vi "Channel Subpanel.vi"() -> ()   [LabVIEW 2021, in "CIF Manager UI.lvlib"]
uses:
  CIF Manager UI.lvlib
  CIFManagerUI Class/Typedef/Channel Connection.ctl
  CIFManagerUI Class/Typedef/Class Data for Manager SubPanel.ctl
  <vilib>/gRPC/LabVIEW gRPC Library/Shared/grpcId.ctl
  <vilib>/CIF Foundation/CIF Core/CIFUI/Typedef/Core UI References.ctl
  <vilib>/CIF Foundation/CIF Core/CIFUI/Typedef/Run Listen Button.ctl
  <vilib>/CIF Foundation/CIF Core/CIFUI/Typedef/SubPanel Events.ctl
  <vilib>/CIF Foundation/CIF Core/CIFUI/Typedef/New Connection Event Data.ctl
  <vilib>/CIF Foundation/CIF Core/CIFUI/Typedef/New Connection Plugin Event Data.ctl
  CIFManagerUI Class/Typedef/Core Manager UI References.ctl
  CIFManagerUI Class/Typedef/New Plugin.ctl
  CIFManagerUI Class/Typedef/CIF_Manager_UI_Tab.ctl
  CIFManagerUI Class/CIF_Manager_UI.lvclass/CIF_Manager_UI.ctl
  <vilib>/CIF Foundation/CIF Core/CIFUI/CIF_UI.lvclass/CIF_UI.ctl
  <vilib>/CIF Foundation/CIF Core/CIFUI/Typedef/Direction to Include.ctl
  <vilib>/CIF Foundation/CIF Utilities/DataTypes/Typedef/Endian.ctl
  <vilib>/CIF Foundation/CIF Core/CIFUI/Typedef/Force Channel.ctl
  <vilib>/CIF Foundation/CIF Core/CIFUI/Utilities/Get Human Readable Error.vi
  <vilib>/CIF Foundation/CIF Utilities/Errors/Append Error Location.vi
  <vilib>/CIF Foundation/CIF Core/CIFUI/Accessors/Read Instrument Studio.vi
  CIFManagerUI Class/CIF_Manager_UI.lvclass
  C:/Program Files/National Instruments/LabVIEW 2021/vi.lib/CIF Foundation/CIF Core/CIFUI/CIF_UI.lvclass
  <vilib>/CIF Foundation/CIF Core/CIFUI/UI Helpers/UI Element Update/Empty Tree by Reference.vi
  CIFManagerUI Class/Manager Functions/SubVIs/Initialize Manager Tab by Reference.vi
  <vilib>/CIF Foundation/CIF Utilities/Errors/Human Readable Error Message.vi
  <vilib>/CIF Foundation/CIF Core/CIFUI/CIF_UI.lvclass
  <vilib>/CIF Foundation/CIF Utilities/DataTypes/DataTypes_CIF_U.lvlib
  <vilib>/gRPC/LabVIEW gRPC Library/grpc-lvsupport-release.lvlib
panel:
  in  "Class Data for Manager SubPanel":T1
  in  "String Force":string
  in  "Force Active":bool
  in  "I64 Force":i64
  in  "U64 Force":u64
  in  "Double Force":dbl
  in  "Forced Data":string
  in  "Channel":string
  in  "Force Channel":bool
  in  "Link Channel":bool
  in  "Connection":T6
  in  "Publisher Channels":string(tree)
  in  "Subscriber Channels":string(tree)
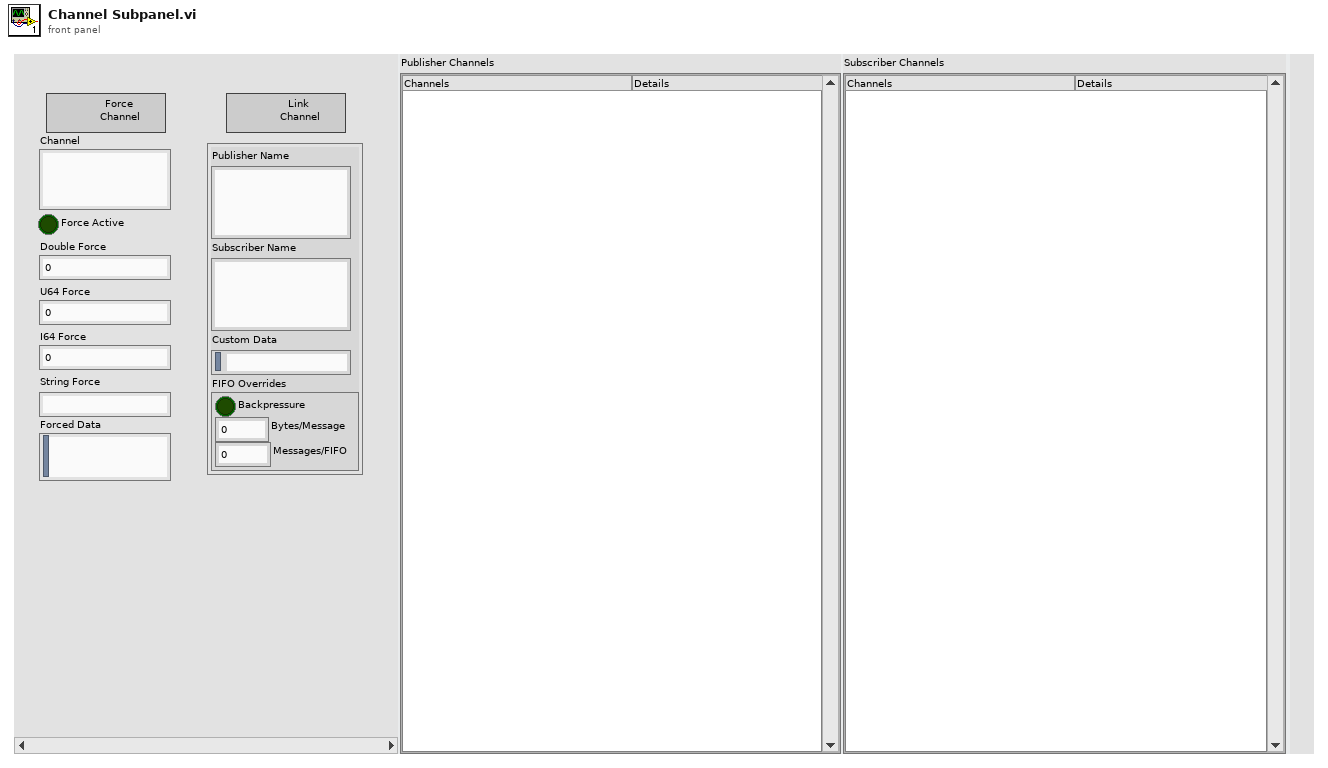
[diagram p1: front panel]
types:
  T1 = typedef "CIF_Manager_UI.lvclass/Class Data for Manager SubPanel.ctl" = cluster{"Class Data for SubPanel":cluster{"IP Address":string, "Manager gRPC ID":T2, "Server Certificate File (.crt)":path, "Connected":bool, "Manager Connection":bool, "Core UI References":T3, "Subpanel Events":T4}, "Manager UI References":T5}
  T2 = typedef "grpc-lvsupport-release.lvlib/grpcId.ctl" = u64
  T3 = typedef "CIF_UI.lvclass/Core UI References.ctl" = cluster{"Plugin Status":refnum<vi>, "Plugin Status Valid":bool, "Connection":refnum<vi>, "Connection Valid":bool, "Exit":refnum<vi>, "Exit Valid":bool, "Run Listen":refnum<vi>, "Run Listen Valid":bool, "Clear Local Error":refnum<vi>, "Clear Local Error Valid":bool, "Local Error":refnum<vi>, "Local Error Valid":bool}
  T4 = typedef "CIF_UI.lvclass/SubPanel Events.ctl" = cluster{"Clear Local Error":refnum<user-event>, "Shutdown":refnum<user-event>, "gRPC Connection":refnum<user-event>, "Plugin Connection":refnum<user-event>}
  T5 = typedef "CIF_Manager_UI.lvclass/Core Manager UI References.ctl" = cluster{"Discovered Plugins":refnum<vi>, "Discovered Plugins Valid":bool, "Loaded Plugins":refnum<vi>, "Loaded Plugins Valid":bool, "Publisher Channels":refnum<vi>, "Publisher Channels Valid":bool, "Subscriber Channels":refnum<vi>, "Subscriber Channels Valid":bool, "Channel Connection":refnum<vi>, "Channel Connection Valid":bool, "New Plugin Load":refnum<vi>, "New Plugin Load Valid":bool, "Errors":refnum<vi>, "Errors Valid":bool, "Plugin to Abort":refnum<vi>, "Plugin to Abort Valid":bool, "CIF Manager Tab":refnum<vi>, "Manger Tab Valid":bool, "System Errors":refnum<vi>, "System Errors Valid":bool, "Plugin Selection":refnum<vi>, "Plugin Selection Valid":bool}
  T6 = typedef "CIF_Manager_UI.lvclass/Channel Connection.ctl" = cluster{"Publisher Name":string, "Subscriber Name":string, "Custom Data":string, "FIFO Overrides":cluster{"Backpressure":bool, "Bytes/Message":u32, "Messages/FIFO":u32}}
  T7 = typedef "CIF_UI.lvclass/Direction to Include.ctl" = enum16{"All", "Subscriber", "Publisher"}
  T8 = enum16{"big-endian, network order", "native, host order", "little-endian"}
  T9 = typedef "DataTypes_CIF_U.lvlib/Endian.ctl" = enum16{"Little Endian", "Big Endian"}
  T10 = typedef "CIF_UI.lvclass/Force Channel.ctl" = cluster{"channel_name":string, "force":bool, "force_data":string}
  T11 = typedef "CIFCoreChannel_client.lvlib/cif_management_common_Channel.ctl" = cluster{"name":string, "direction":T12, "type":string, "custom_config":u8[], "connected":bool, "connected_name":string, "forced":bool, "channel_pattern":T13}
  T12 = typedef "CIFCoreChannel_client.lvlib/cif_management_common_ChannelDirection.ctl" = enum32{"CHANNELDIRECTION_UNKNOWN", "CHANNELDIRECTION_PUBLISHER", "CHANNELDIRECTION_SUBSCRIBER"}
  T13 = typedef "CIFCoreChannel_client.lvlib/cif_management_common_ChannelPattern.ctl" = enum32{"CHANNELPATTERN_UNKNOWN", "CHANNELPATTERN_TAG", "CHANNELPATTERN_FIFO", "CHANNELPATTERN_MULTIFIFO", "CHANNELPATTERN_BACKPRESSUREFIFO"}
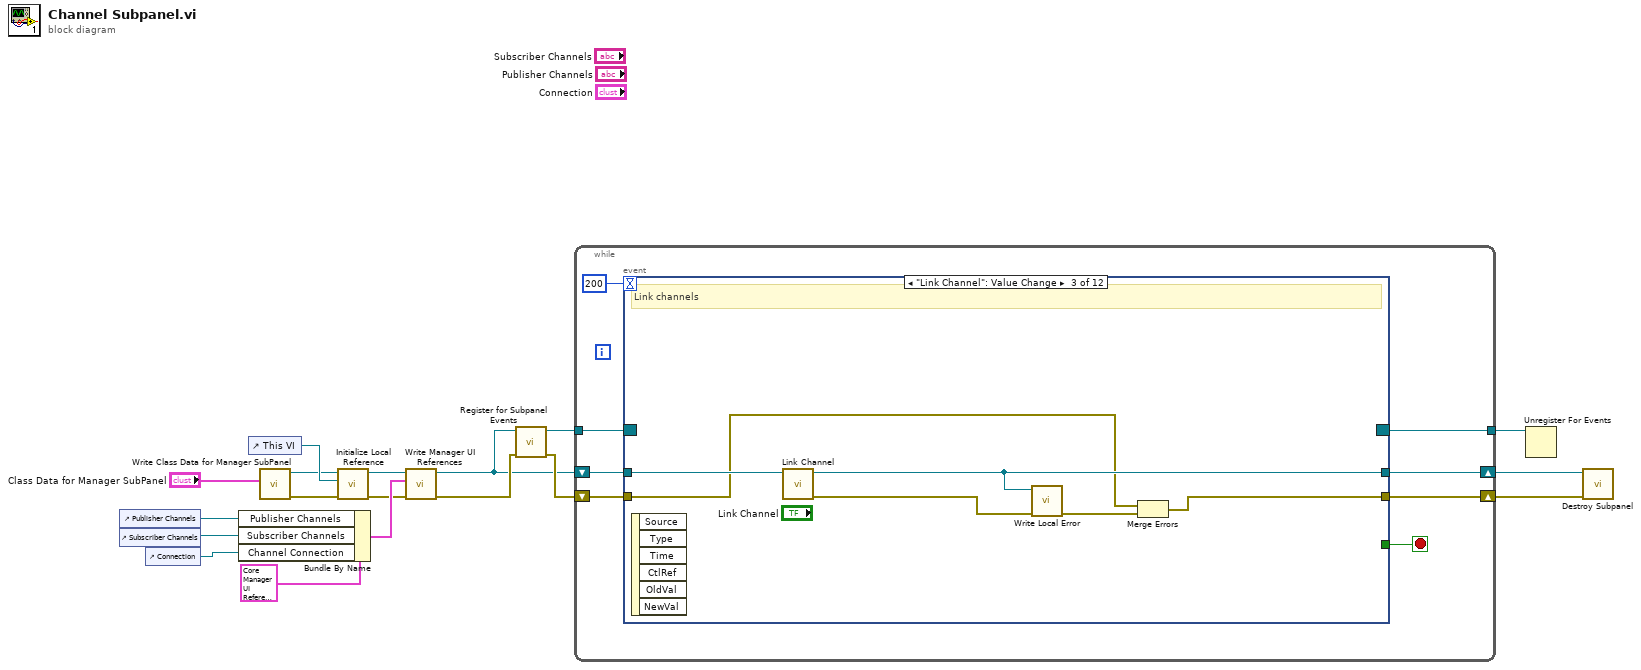
[diagram p0: block diagram]
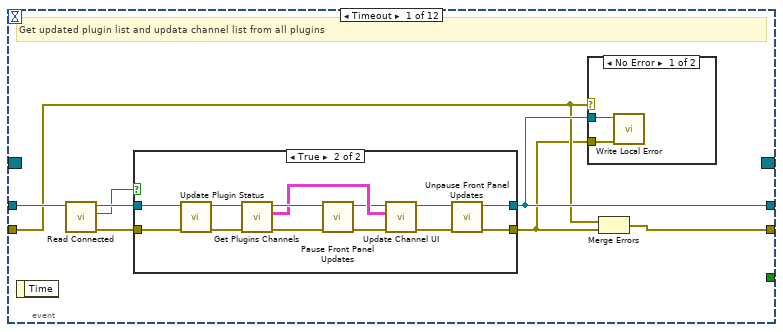
[diagram p2: hidden frame]
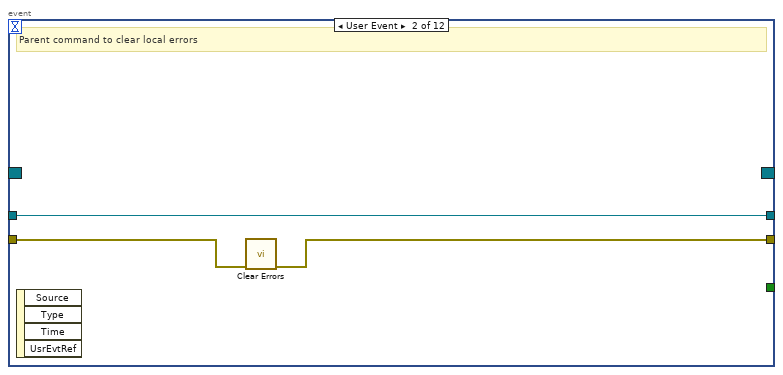
[diagram p5: hidden frame]
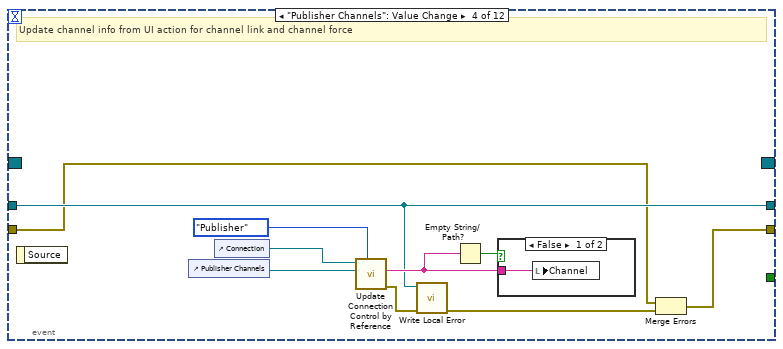
[diagram p6: hidden frame]
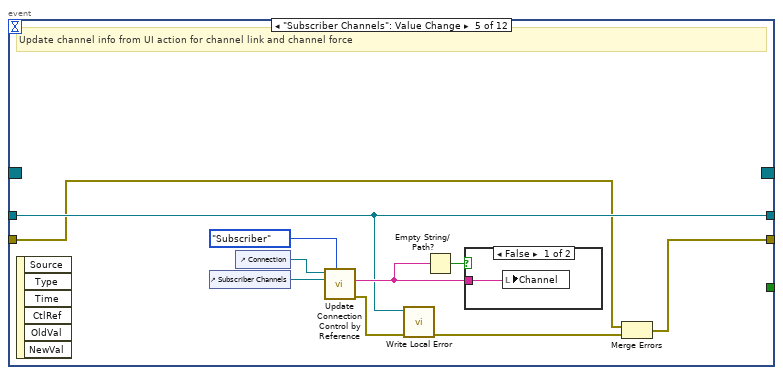
[diagram p8: hidden frame]
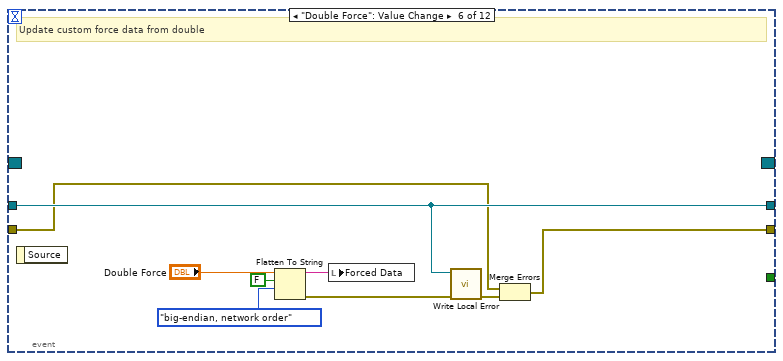
[diagram p10: hidden frame]
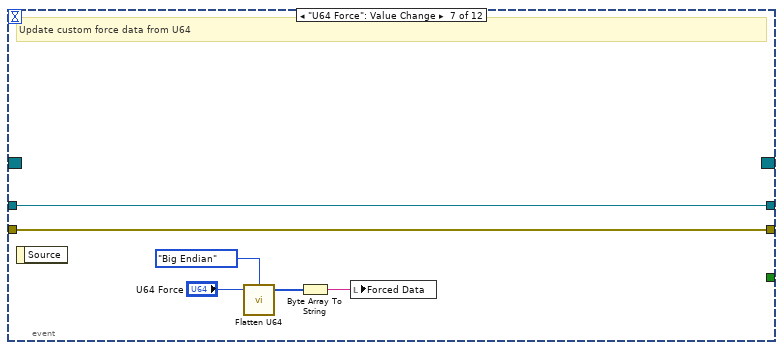
[diagram p11: hidden frame]
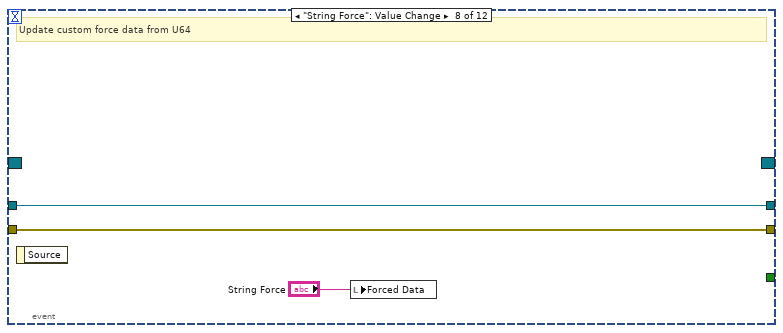
[diagram p12: hidden frame]
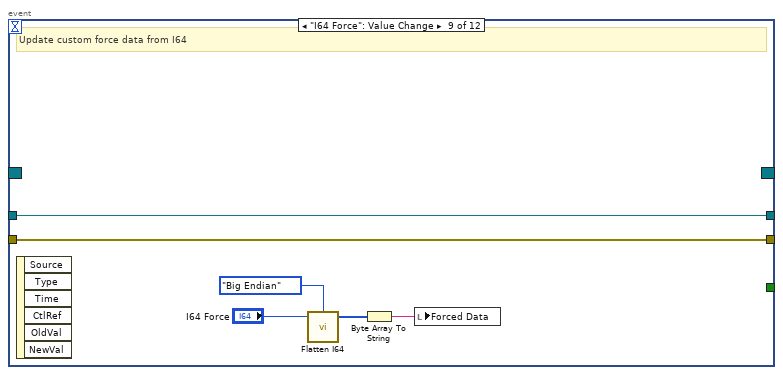
[diagram p13: hidden frame]
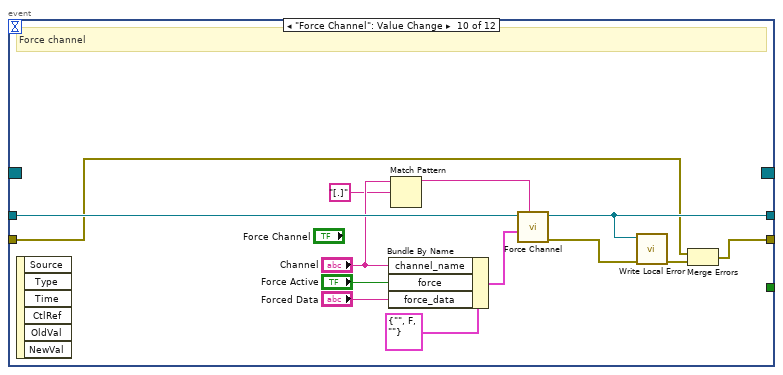
[diagram p14: hidden frame]
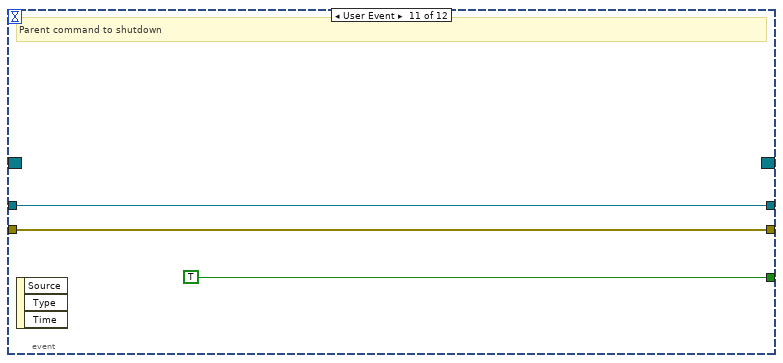
[diagram p15: hidden frame]
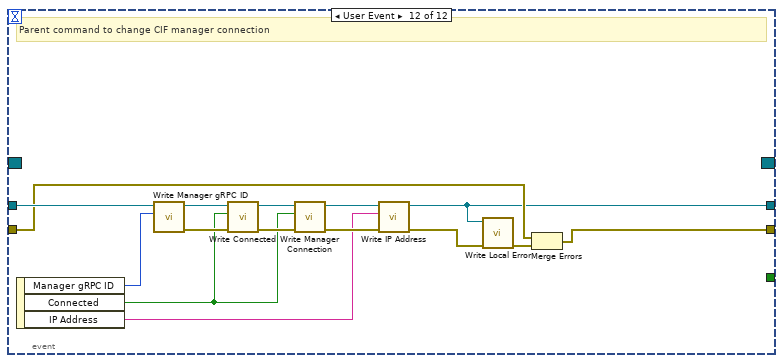
[diagram p16: hidden frame]
diagram:
  n1 = control-ref of="Publisher Channels"() -> (w18:refnum<vi>)
  n2 = control-ref of="Subscriber Channels"() -> (w17:refnum<vi>)
  n3 = control-ref of="Connection"() -> (w16:refnum<vi>)
  n4 = Bundle By Name(cluster=T5 {"Discovered Plugins"=refnum, "Discovered Plugins Valid"=FALSE, "Loaded Plugins"=refnum, "Loaded Plugins Valid"=FALSE, "Publisher Channels"=refnum, "Publisher Channels Valid"=FALSE, "Subscriber Channels"=refnum, "Subscriber Channels Valid"=FALSE, "Channel Connection"=refnum, "Channel Connection Valid"=FALSE, "New Plugin Load"=refnum, "New Plugin Load Valid"=FALSE, "Errors"=refnum, "Errors Valid"=FALSE, "Plugin to Abort"=refnum, "Plugin to Abort Valid"=FALSE, "CIF Manager Tab"=refnum, "Manger Tab Valid"=FALSE, "System Errors"=refnum, "System Errors Valid"=FALSE, "Plugin Selection"=refnum, "Plugin Selection Valid"=FALSE} ("Manager UI References"), "Publisher Channels"=w18, "Subscriber Channels"=w17, "Channel Connection"=w16) -> (w9:T5)
  n5 = control-ref of="This VI"() -> (w13:refnum<vi>)
  n6 = call "Write Class Data for Manager SubPanel.vi"("Class Data for Manager SubPanel"="Class Data for Manager SubPanel") -> ("error out"=w4:errorcluster, "CIF_Manager_UI out"=w3:refnum<class "CIF_Manager_UI.lvclass">)  [unwired: 9 in]
  n7 = call <vilib>:"Initialize Local Reference.vi"("error in (no error)"=w4, "This VI"=w13, "CIF_UI in"=w3) -> ("error out"=w7:errorcluster, "CIF_UI out"=w8:refnum<class "CIF_Manager_UI.lvclass">)  [unwired: 7 in]
  n8 = call "Write Manager UI References.vi"("error in (no error)"=w7, "Manager UI References"=w9, "CIF_UI in"=w8) -> ("error out"=w6:errorcluster, "CIF_UI out"=w5:refnum<class "CIF_Manager_UI.lvclass">)  [unwired: 7 in]
  n9 = call <vilib>:"Register for Subpanel Events.vi"("error in (no error)"=w6, "CIF_UI in"=w5) -> ("error out"=w14:errorcluster, "Event Registration Refnum"=w15:refnum<event-registration>)  [unwired: 8 in]
  n10 = while {
    tunnel: w15 -> [w25]
    shift-right: [w21] -> w12
    shift-left: w5 -> [w23]
    shift-right: [w19] -> w10
    shift-left: w14 -> [w22]
    tunnel: [w20] -> w11
    stop <- w24 stop-if-true
    n11 = event shown="[2] \"Link Channel\": Value Change" {
      selector: w25 -> [_ _ _ _ _ _ _ _ _ _ _ _]
      dyn-events: [_ _ _ _ _ _ _ _ _ _ _ _] -> w20
      timeout: 200 -> [_ _ _ _ _ _ _ _ _ _ _ _]
      tunnel: [_ _ _ _ _ _ _ _ _ _ TRUE _] -> w24
      tunnel: w23 -> [w31 w52 w60 w64 w75 w85 w97 w100 w102 w119 w121 w131]
      tunnel: w22 -> [w29 w54 w56 w62 w72 w84 w96 w99 w101 w107 w120 w124]
      tunnel: [w27 w53 w55 w61 w73 w83 w96 w99 w101 w108 w120 w125] -> w19
      tunnel: [w30 w52 w59 w64 w75 w85 w97 w100 w102 w111 w121 w123] -> w21
      event Timeout {
        # "Get updated plugin list and updata channel list from all plugins"
        n12 = event-data() -> ()  [unwired: 1 in, 1 out]
        n13 = call <vilib>:"Read Connected.vi"("CIF_UI in"=w31) -> ("error out"=w33:errorcluster, "Connected"=w32:bool, "CIF_UI out"=w34:refnum<class "CIF_Manager_UI.lvclass">)  [unwired: 8 in]
        n14 = case shown="True" w32 {
          tunnel: w33 -> [w37 w44]
          tunnel: [w37 w51] -> w28
          tunnel: w34 -> [w38 w45]
          tunnel: [w38 w50] -> w30
          frame False {
          }
          frame True {
            n15 = call <vilib>:"Update Plugin Status.vi"("error in (no error)"=w44, "CIF_UI in"=w45) -> ("error out"=w48:errorcluster, "CIF_UI out"=w49:refnum<class "CIF_Manager_UI.lvclass">)  [unwired: 8 in]
            n16 = call <vilib>:"Get Plugins Channels.vi"("error in (no error)"=w48, "CIF_UI in"=w49) -> ("error out"=w40:errorcluster, "Channels"=w42:T11[][], "CIF_UI out"=w43:refnum<class "CIF_Manager_UI.lvclass">)  [unwired: 6 in, 1 out]
            n17 = call <vilib>:"Pause Front Panel Updates.vi"("error in (no error)"=w40, "CIF_UI in"=w43) -> ("error out"=w39:errorcluster, "CIF_UI out"=w41:refnum<class "CIF_Manager_UI.lvclass">)  [unwired: 8 in]
            n18 = call "Update Channel UI.vi"("error in (no error)"=w39, "Channels"=w42, "CIF_UI in"=w41) -> ("error out"=w46:errorcluster, "CIF_UI out"=w47:refnum<class "CIF_Manager_UI.lvclass">)  [unwired: 7 in]
            n19 = call <vilib>:"Unpause Front Panel Updates.vi"("error in (no error)"=w46, "CIF_UI in"=w47) -> ("error out"=w51:errorcluster, "CIF_UI out"=w50:refnum<class "CIF_Manager_UI.lvclass">)  [unwired: 8 in]
          }
        }
        n20 = case shown="No Error" w29 {
          tunnel: w28 -> [w36 _]
          tunnel: w30 -> [w35 _]
          frame No Error {
            n21 = call <vilib>:"Write Local Error.vi"("error in (no error)"=w36, "CIF_UI in"=w35) -> ()  [unwired: 9 in, 1 out]
          }
          frame Error {
          }
        }
        n22 = Merge Errors(w29, w28) -> (w27:errorcluster)
      }
      event User Event {
        # "Parent command to clear local errors"
        n23 = event-data() -> ()  [unwired: 1 in, 4 out]
        n24 = call <vilib>:"Clear Errors.vi"("error in (no error)"=w54) -> ("error out"=w53:errorcluster)  [unwired: 5 in, 1 out]
      }
      event "Link Channel": Value Change {
        # "Link channels"
        n25 = event-data() -> ()  [unwired: 1 in, 6 out]
        n26 = call "Link Channel.vi"("CIF_UI in"=w60) -> ("error out"=w58:errorcluster, "CIF_UI out"=w59:refnum<class "CIF_Manager_UI.lvclass">)  [unwired: 9 in]
        n27 = call <vilib>:"Write Local Error.vi"("error in (no error)"=w58, "CIF_UI in"=w59) -> ("error out"=w57:errorcluster)  [unwired: 9 in]
        n28 = Merge Errors(w56, w57) -> (w55:errorcluster)
      }
      event "Publisher Channels": Value Change {
        # "Update channel info from UI action for channel link and channel force"
        n29 = event-data() -> ()  [unwired: 1 in, 1 out]
        n30 = control-ref of="Publisher Channels"() -> (w68:refnum<vi>)
        n31 = control-ref of="Connection"() -> (w69:refnum<vi>)
        n32 = call "Update Connection Control by Reference.vi"("Direction to Include"=Direction_to_Include."Publisher", "Channels"=w68, "Channel Connection"=w69) -> ("error out"=w65:errorcluster, "Channel Name"=w66:string)  [unwired: 7 in]
        n33 = call <vilib>:"Write Local Error.vi"("error in (no error)"=w65, "CIF_UI in"=w64) -> ("error out"=w63:errorcluster)  [unwired: 9 in]
        n34 = Empty String/Path?(string/path=w66) -> (empty?=w67:bool)
        n35 = case shown="False" w67 {
          tunnel: w66 -> [w71 _]
          frame False {
            n36 = local write "Channel"(w71) -> ()
          }
          frame True {
          }
        }
        n37 = Merge Errors(w62, w63) -> (w61:errorcluster)
      }
      event "Subscriber Channels": Value Change {
        # "Update channel info from UI action for channel link and channel force"
        n38 = event-data() -> ()  [unwired: 1 in, 6 out]
        n39 = control-ref of="Subscriber Channels"() -> (w79:refnum<vi>)
        n40 = control-ref of="Connection"() -> (w80:refnum<vi>)
        n41 = call "Update Connection Control by Reference.vi"("Direction to Include"=Direction_to_Include."Subscriber", "Channels"=w79, "Channel Connection"=w80) -> ("error out"=w76:errorcluster, "Channel Name"=w77:string)  [unwired: 7 in]
        n42 = call <vilib>:"Write Local Error.vi"("error in (no error)"=w76, "CIF_UI in"=w75) -> ("error out"=w74:errorcluster)  [unwired: 9 in]
        n43 = Empty String/Path?(string/path=w77) -> (empty?=w78:bool)
        n44 = case shown="False" w78 {
          tunnel: w77 -> [w82 _]
          frame False {
            n45 = local write "Channel"(w82) -> ()
          }
          frame True {
          }
        }
        n46 = Merge Errors(w72, w74) -> (w73:errorcluster)
      }
      event "Double Force": Value Change {
        # "Update custom force data from double"
        n47 = event-data() -> ()  [unwired: 1 in, 1 out]
        n48 = Flatten To String(anything="Double Force", prepend array or string size? (T)=FALSE, byte order (0:big-endian, network order)=T8."big-endian, network order") -> (data string=w88:string, error out=w86:errorcluster)  [unwired: 1 in, 1 out]
        n49 = local write "Forced Data"(w88) -> ()
        n50 = call <vilib>:"Write Local Error.vi"("error in (no error)"=w86, "CIF_UI in"=w85) -> ("error out"=w87:errorcluster)  [unwired: 9 in]
        n51 = Merge Errors(w84, w87) -> (w83:errorcluster)
      }
      event "U64 Force": Value Change {
        # "Update custom force data from U64"
        n52 = event-data() -> ()  [unwired: 1 in, 1 out]
        n53 = call <vilib>:"Flatten U64.vi"("U64"="U64 Force", "Endian"=Endian."Big Endian") -> ("Flat Data"=w93:u8[])  [unwired: 3 in]
        n54 = Byte Array To String(unsigned byte array=w93) -> (string=w94:string)
        n55 = local write "Forced Data"(w94) -> ()
      }
      event "String Force": Value Change {
        # "Update custom force data from U64"
        n56 = event-data() -> ()  [unwired: 1 in, 1 out]
        n57 = local write "Forced Data"("String Force") -> ()
      }
      event "I64 Force": Value Change {
        # "Update custom force data from I64"
        n58 = event-data() -> ()  [unwired: 1 in, 6 out]
        n59 = call <vilib>:"Flatten I64.vi"("I64"="I64 Force", "Endian"=Endian."Big Endian") -> ("Flat Data"=w105:u8[])  [unwired: 3 in]
        n60 = Byte Array To String(unsigned byte array=w105) -> (string=w106:string)
        n61 = local write "Forced Data"(w106) -> ()
      }
      event "Force Channel": Value Change {
        # "Force channel"
        n62 = event-data() -> ()  [unwired: 1 in, 6 out]
        n63 = Bundle By Name(cluster=T10 {"channel_name"="", "force"=FALSE, "force_data"=""} ("Force Channel"), "channel_name"="Channel", "force"="Force Active", "force_data"="Forced Data") -> (w117:T10)
        n64 = Match Pattern(string="Channel", regular expression="[.]") -> (before substring=w112:string)  [unwired: 1 in, 3 out]
        n65 = call <vilib>:"Force Channel.vi"("Plugin Name"=w112, "Force Channel"=w117, "CIF_Plugin_UI in"=w119) -> ("error out"=w110:errorcluster, "CIF_Plugin_UI out"=w111:refnum<class "CIF_Manager_UI.lvclass">)  [unwired: 6 in, 1 out]
        n66 = call <vilib>:"Write Local Error.vi"("error in (no error)"=w110, "CIF_UI in"=w111) -> ("error out"=w109:errorcluster)  [unwired: 9 in]
        n67 = Merge Errors(w107, w109) -> (w108:errorcluster)
      }
      event User Event {
        # "Parent command to shutdown"
        n68 = event-data() -> ()  [unwired: 1 in, 3 out]
      }
      event User Event {
        # "Parent command to change CIF manager connection"
        n69 = event-data() -> ("Manager gRPC ID"=w128:T2, "Connected"=w129:bool, "IP Address"=w130:string)  [unwired: 1 in]
        n70 = call <vilib>:"Write Manager gRPC ID.vi"("gRPCid"=w128, "CIF_UI in"=w131) -> ("error out"=w133:errorcluster, "CIF_UI out"=w132:refnum<class "CIF_Manager_UI.lvclass">)  [unwired: 8 in]
        n71 = call <vilib>:"Write Connected.vi"("error in (no error)"=w133, "Connected"=w129, "CIF_UI in"=w132) -> ("error out"=w135:errorcluster, "CIF_UI out"=w134:refnum<class "CIF_Manager_UI.lvclass">)  [unwired: 7 in]
        n72 = call <vilib>:"Write Manager Connection.vi"("error in (no error)"=w135, "Manager Connection"=w129, "CIF_UI in"=w134) -> ("error out"=w137:errorcluster, "CIF_UI out"=w136:refnum<class "CIF_Manager_UI.lvclass">)  [unwired: 7 in]
        n73 = call <vilib>:"Write IP Address.vi"("error in (no error)"=w137, "IP Address"=w130, "CIF_UI in"=w136) -> ("error out"=w126:errorcluster, "CIF_UI out"=w123:refnum<class "CIF_Manager_UI.lvclass">)  [unwired: 7 in]
        n74 = call <vilib>:"Write Local Error.vi"("error in (no error)"=w126, "CIF_UI in"=w123) -> ("error out"=w127:errorcluster)  [unwired: 9 in]
        n75 = Merge Errors(w124, w127) -> (w125:errorcluster)
      }
    }
  }
  n76 = Unregister For Events(event registration refnum=w11) -> ()  [unwired: 1 in, 1 out]
  n77 = call <vilib>:"Destroy Subpanel.vi"("error in (no error)"=w10, "CIF_UI in"=w12) -> ()  [unwired: 8 in, 2 out]
